vi "UHR-Fleezers Control (host) -Mau_stepping.vi"(0 "Tab Control":T5(tab)) -> ()   [LabVIEW 2013] (continued)
            n1103 = case shown="True" "Move Trap After?" {
              frame False {
              }
              frame True {
                n1104 = property on="Trap Delta (MHz)" class="DigNum (strict)"("Val(Sgnl)"="Dip Trap Delta 2 (MHz)") -> ()  [unwired: 2 in, 2 out]
              }
            }
          }
          frame #3 {
            n1105 = case shown="True" "Green ON After?" {
              frame False {
              }
              frame True {
                n1106 = property on="Green Laser ON/Interlacing" class="Bool (strict)"("Val(Sgnl)"=TRUE ("Value (Signaling)")) -> ()  [unwired: 2 in, 2 out]
              }
            }
          }
          frame #4 {
            n1107 = Wait (ms)(milliseconds to wait=u32 500) -> ()  [unwired: 1 out]
          }
          frame #5 {
            n1108 = case shown="True" "Save Data After?" {
              frame False {
              }
              frame True {
                n1109 = property on="Start Saving" class="Bool (strict)"("Val(Sgnl)"=TRUE ("Value (Signaling)")) -> ()  [unwired: 2 in, 2 out]
              }
            }
          }
        }
      }
      event "Profile": Value Change {
        n1110 = event-data() -> ()  [unwired: 1 in, 5 out]
        n1111 = flat-sequence {
          frame #0 {
            w1714 = 0.0 ("element")
            n1112 = Build Array(w1714, "Y change (mm)", w1714) -> ()  [unwired: 1 out]
          }
          frame #1 {
            # "stop saving"
            n1113 = local write "Stop Saving"(TRUE ("Stop Saving")) -> ()
            n1114 = local write "Stage Moving"(FALSE ("Stage Moving")) -> ()
          }
        }
      }
      event "Got ADig bead": Value Change {
        n1115 = event-data() -> ()  [unwired: 1 in, 5 out]
        n1116 = property on="Move Cap. 1 (DNA Top)" class="Bool (strict)"("Val(Sgnl)"=TRUE ("Value (Signaling)")) -> ()  [unwired: 2 in, 2 out]
        n1117 = property on="Inject Top:" class="Bool (strict)"("Val(Sgnl)"=FALSE ("Value (Signaling)")) -> ()  [unwired: 2 in, 2 out]
      }
      event "Got DNA bead": Value Change {
        n1118 = event-data() -> ()  [unwired: 1 in, 5 out]
        n1119 = property on="Cal/Data Acq. Spot" class="Bool (strict)"("Val(Sgnl)"=TRUE ("Value (Signaling)")) -> ()  [unwired: 2 in, 2 out]
        n1120 = property on="Main:" class="Bool (strict)"("Val(Sgnl)"=FALSE ("Value (Signaling)")) -> ()  [unwired: 2 in, 2 out]
      }
      event "Take Stepping Data": Value Change {
        n1121 = event-data() -> ()  [unwired: 1 in, 5 out]
        n1122 = local read "Save ave N"() -> (w1732:dbl)
        n1123 = flat-sequence {
          tunnel: w1732 -> [w1734]
          tunnel: [w1734] -> w1727
          tunnel: [w1736] -> w1728
          tunnel: w1727 -> [w1736]
          tunnel: [w1738] -> w1729
          tunnel: w1728 -> [w1738]
          tunnel: [w1741] -> w1730
          tunnel: w1729 -> [w1741]
          tunnel: [w1743] -> w1731
          tunnel: w1730 -> [w1743]
          tunnel: [w1745] -> w1725
          tunnel: w1731 -> [w1745]
          tunnel: w1725 -> [w1748]
          tunnel: [w1748] -> w1724
          tunnel: w1724 -> [w1749]
          tunnel: [w1749] -> w1726
          tunnel: w1726 -> [w1755]
          frame #0 {
            n1124 = property on="Save ave N" class="DigNum (strict)"("Val(Sgnl)"="Save ave factor") -> ()  [unwired: 2 in, 2 out]
          }
          frame #1 {
            n1125 = Wait (ms)(milliseconds to wait=u32 100) -> ()  [unwired: 1 out]
          }
          frame #2 {
            n1126 = local read "Offset 2 Start (MHz)"() -> (w1740:dbl)
            n1127 = property on="Saved AOD Raster Scan Parameter Sets" class="Arr (strict)"("Index Values"=u32[] [2]) -> ()  [unwired: 2 in, 2 out]
            n1128 = property on="Trap Delta (MHz)" class="DigNum (strict)"("Val(Sgnl)"=w1740) -> ()  [unwired: 2 in, 2 out]
          }
          frame #3 {
            n1129 = property on="Load parameters" class="Bool (strict)"("Val(Sgnl)"=TRUE ("Value (Signaling)")) -> ()  [unwired: 2 in, 2 out]
          }
          frame #4 {
            n1130 = Wait (ms)(milliseconds to wait=u32 100) -> ()  [unwired: 1 out]
          }
          frame #5 {
            n1131 = property on="Trap Raster Scan" class="Bool (strict)"("Val(Sgnl)"=TRUE ("Value (Signaling)")) -> ()  [unwired: 2 in, 2 out]
          }
          frame #6 {
            n1132 = Wait (ms)(milliseconds to wait=u32 1000) -> ()  [unwired: 1 out]
          }
          frame #7 {
            n1133 = while {
              stop <- w1752 stop-if-true
              n1134 = local read "Raster Scanning..."() -> (w1754:bool)
              n1135 = local read "Saving..."() -> (w1753:bool)
              n1136 = Not(x=w1753) -> (.not. x?=w1750:bool)
              n1137 = Not(x=w1754) -> (.not. x?=w1751:bool)
              n1138 = And(x=w1751, y=w1750) -> (x .and. y?=w1752:bool)
            }
          }
          frame #8 {
            n1139 = property on="Save ave N" class="DigNum (strict)"("Val(Sgnl)"=w1755) -> ()  [unwired: 2 in, 2 out]
          }
        }
      }
      event "Step Size (nm)": Value Change {
        n1140 = event-data() -> ()  [unwired: 1 in, 5 out]
        n1141 = flat-sequence {
          frame #0 {
            n1142 = property on="Saved AOD Raster Scan Parameter Sets" class="Arr (strict)"("Index Values"=u32[] [1]) -> ()  [unwired: 2 in, 2 out]
          }
          frame #1 {
            n1143 = Multiply(x="N Steps", y="Step Size (nm)") -> (x*y=w1757:dbl)
            n1144 = property on="Scan Speed AOD (nm/s) 2" class="DigNum (strict)"("Value"="Step Size (nm)") -> ()  [unwired: 2 in, 2 out]
            n1145 = property on="Step Size AOD (nm) 2" class="DigNum (strict)"("Value"="Step Size (nm)") -> ()  [unwired: 2 in, 2 out]
            n1146 = property on="Scan Range AOD (nm) 2" class="DigNum (strict)"("Value"=w1757) -> ()  [unwired: 2 in, 2 out]
          }
        }
      }
      event "Take Detection Laser\nImage": Value Change {
        n1147 = event-data() -> ()  [unwired: 1 in, 5 out]
        n1148 = flat-sequence {
          tunnel: [w1785] -> w1775
          tunnel: [w1784] -> w1768
          tunnel: [w1783] -> w1760
          tunnel: [w1788] -> w1776
          tunnel: w1775 -> [w1788]
          tunnel: [w1787] -> w1769
          tunnel: w1768 -> [w1787]
          tunnel: [w1786] -> w1761
          tunnel: w1760 -> [w1786]
          tunnel: [w1792] -> w1777
          tunnel: w1776 -> [w1792]
          tunnel: [w1791] -> w1770
          tunnel: w1769 -> [w1791]
          tunnel: [w1790] -> w1762
          tunnel: w1761 -> [w1790]
          tunnel: [w1798] -> w1778
          tunnel: w1777 -> [w1798]
          tunnel: [w1797] -> w1771
          tunnel: w1770 -> [w1797]
          tunnel: [w1796] -> w1763
          tunnel: w1762 -> [w1796]
          tunnel: [w1802] -> w1779
          tunnel: w1778 -> [w1802]
          tunnel: [w1801] -> w1772
          tunnel: w1771 -> [w1801]
          tunnel: [w1800] -> w1764
          tunnel: w1763 -> [w1800]
          tunnel: [w1806] -> w1780
          tunnel: w1779 -> [w1806]
          tunnel: [w1805] -> w1773
          tunnel: w1772 -> [w1805]
          tunnel: [w1804] -> w1765
          tunnel: w1764 -> [w1804]
          tunnel: [w1810] -> w1781
          tunnel: w1780 -> [w1810]
          tunnel: [w1809] -> w1774
          tunnel: w1773 -> [w1809]
          tunnel: [w1808] -> w1766
          tunnel: w1765 -> [w1808]
          tunnel: w1781 -> [w1816]
          tunnel: w1774 -> [w1815]
          tunnel: [w1813] -> w1767
          tunnel: w1766 -> [w1813]
          tunnel: w1767 -> [w1817]
          frame #0 {
            n1149 = local read "Green Laser ON/Interlacing"() -> (w1785:bool)
            n1150 = local read "Green laser mode"() -> (w1784:enum32{"Laser ON", "Laser OFF", "Interlace"})
            n1151 = local read "Green FB On/Off"() -> (w1783:bool)
          }
          frame #1 {
            n1152 = property on="Green FB On/Off" class="Bool (strict)"("Val(Sgnl)"=FALSE ("Value (Signaling)")) -> ()  [unwired: 2 in, 2 out]
          }
          frame #2 {
            n1153 = property on="Green Laser ON/Interlacing" class="Bool (strict)"("Val(Sgnl)"=TRUE ("Value (Signaling)")) -> ()  [unwired: 2 in, 2 out]
            n1154 = property on="Flip Green Filter" class="Bool (strict)"("Val(Sgnl)"=TRUE ("Value (Signaling)")) -> ()  [unwired: 2 in, 2 out]
            n1155 = property on="Green laser mode" class="RadioBtnsControl (strict)"("Val(Sgnl)"=enum32{"Laser ON", "Laser OFF", "Interlace"}."Laser ON" ("Value (Signaling)")) -> ()  [unwired: 2 in, 2 out]
          }
          frame #3 {
            n1156 = Wait (ms)(milliseconds to wait=u32 500) -> ()  [unwired: 1 out]
          }
          frame #4 {
            n1157 = property on="Confocal Image" class="Bool (strict)"("Val(Sgnl)"=TRUE ("Value (Signaling)")) -> ()  [unwired: 2 in, 2 out]
          }
          frame #5 {
            n1158 = Wait (ms)(milliseconds to wait=u32 2000) -> ()  [unwired: 1 out]
          }
          frame #6 {
            n1159 = while {
              stop <- w1811 stop-if-true
              n1160 = local read "Saving..."() -> (w1812:bool)
              n1161 = Not(x=w1812) -> (.not. x?=w1811:bool)
            }
          }
          frame #7 {
            n1162 = property on="Flip Green Filter" class="Bool (strict)"("Val(Sgnl)"=TRUE ("Value (Signaling)")) -> ()  [unwired: 2 in, 2 out]
            n1163 = property on="Green Laser ON/Interlacing" class="Bool (strict)"("Val(Sgnl)"=w1816) -> ()  [unwired: 2 in, 2 out]
            n1164 = property on="Green laser mode" class="RadioBtnsControl (strict)"("Val(Sgnl)"=w1815) -> ()  [unwired: 2 in, 2 out]
          }
          frame #8 {
            n1165 = property on="Green FB On/Off" class="Bool (strict)"("Val(Sgnl)"=w1817) -> ()  [unwired: 2 in, 2 out]
          }
        }
      }
      event "Stop All": Value Change {
        n1166 = event-data() -> ()  [unwired: 1 in, 5 out]
        n1167 = local read "Stop All"() -> (w1818:bool)
      }
    }
    n1168 = node-c288() -> ()  [unwired: 1 in, 1 out]
  }
  n1169 = node-c288() -> (w76:T24)  [unwired: 4 out]
  n1170 = timed-loop "Mouse control: trap position (AOM deflection), set confocal spot from image" {
    tunnel: [w1820] -> w34
    tunnel: w24 -> [w1819]
    timing: w76 -> [_]
    timing-out: [_] -> w75
    stop <- w1820 stop-if-true
    n1171 = node-c288() -> ()  [unwired: 2 out]
    n1172 = event shown="[0] \"Pane\": Mouse Down" {
      selector: _ -> [_ _]
      dyn-events: _ -> [_ _]
      timeout: _ -> [_ _]
      tunnel: w1819 -> [w1823 _]
      event Mouse Down {
        n1173 = event-data() -> ("Time"=w1825:u32, "Coords"=w1824:T8, "Button"=w1826:u16)  [unwired: 6 out]
        n1174 = case shown="1" w1826 {
          tunnel: w1825 -> [_ _ w1929]
          tunnel: w1824 -> [_ w1863 w1927]
          tunnel: w1823 -> [_ _ w1925]
          frame 0, Default {
          }
          frame 1 {
            n1175 = property on="APD 2" class="ImageControl"() -> ("Displayed Image Position"=w1833:cluster{"Left":i32, "Top":i32})  [unwired: 2 in, 2 out]
            n1176 = property on="APD 1" class="ImageControl"() -> ("Displayed Image Position"=w1862:cluster{"Left":i32, "Top":i32})  [unwired: 2 in, 2 out]
            n1177 = property on="Detection Laser X" class="ImageControl"() -> ("Displayed Image Position"=w1859:cluster{"Left":i32, "Top":i32})  [unwired: 2 in, 2 out]
            n1178 = property on="Detection Laser Y" class="ImageControl"() -> ("Displayed Image Position"=w1858:cluster{"Left":i32, "Top":i32})  [unwired: 2 in, 2 out]
            n1179 = property on="APD 2" class="ImageControl"() -> ("Displayed Image Size"=w1832:cluster{"Width":u32, "Height":u32})  [unwired: 2 in, 2 out]
            n1180 = property on="APD 1" class="ImageControl"() -> ("Displayed Image Size"=w1860:cluster{"Width":u32, "Height":u32})  [unwired: 2 in, 2 out]
            n1181 = property on="Detection Laser X" class="ImageControl"() -> ("Displayed Image Size"=w1861:cluster{"Width":u32, "Height":u32})  [unwired: 2 in, 2 out]
            n1182 = property on="Detection Laser Y" class="ImageControl"() -> ("Displayed Image Size"=w1857:cluster{"Width":u32, "Height":u32})  [unwired: 2 in, 2 out]
            n1183 = Unbundle By Name(w1832) -> ("Width"=w1829:u32, "Height"=w1828:u32)
            n1184 = Unbundle By Name(w1833) -> ("Left"=w1831:i32, "Top"=w1830:i32)
            n1185 = Unbundle By Name(w1860) -> ("Width"=w1854:u32, "Height"=w1853:u32)
            n1186 = Unbundle By Name(w1861) -> ("Width"=w1850:u32, "Height"=w1849:u32)
            n1187 = Unbundle By Name(w1857) -> ("Width"=w1846:u32, "Height"=w1845:u32)
            n1188 = Unbundle By Name(w1862) -> ("Left"=w1856:i32, "Top"=w1855:i32)
            n1189 = Unbundle By Name(w1859) -> ("Left"=w1852:i32, "Top"=w1851:i32)
            n1190 = Unbundle By Name(w1858) -> ("Left"=w1848:i32, "Top"=w1847:i32)
            n1191 = Bundle("Left"=w1831, "Top"=w1830, "Width"=w1829, "Height"=w1828) -> (w1827:T33)  [unwired: 1 in]
            n1192 = Bundle("Left"=w1856, "Top"=w1855, "Width"=w1854, "Height"=w1853) -> (w1844:T33)  [unwired: 1 in]
            n1193 = Bundle("Left"=w1852, "Top"=w1851, "Width"=w1850, "Height"=w1849) -> (w1843:T33)  [unwired: 1 in]
            n1194 = Bundle("Left"=w1848, "Top"=w1847, "Width"=w1846, "Height"=w1845) -> (w1842:T33)  [unwired: 1 in]
            n1195 = Build Cluster Array(w1827, w1844, w1843, w1842) -> (w1841:T34)
            n1196 = for {
              tunnel: w1863 -> [w1874]
              tunnel: w1841 -> [w1875] mode=indexing
              shift-right: [w1872] -> w1839
              shift-left: TRUE -> [w1873]
              shift-right: [w1871] -> w1837
              shift-left: _ -> [w1867]
              shift-right: [w1870] -> w1836
              shift-left: _ -> [w1866]
              shift-right: [w1869] -> w1835
              shift-left: _ -> [w1865]
              shift-right: [w1868] -> w1834
              shift-left: _ -> [w1864]
              n1197 = case shown="True" w1873 {
                selector: w1873 -> [w1880 _]
                tunnel: w1875 -> [_ w1889]
                tunnel: w1874 -> [_ w1887]
                tunnel: [w1880 w1885] -> w1872
                tunnel: [w1879 w1884] -> w1871
                tunnel: [w1878 w1883] -> w1870
                tunnel: [w1877 w1882] -> w1869
                tunnel: [w1876 w1881] -> w1868
                tunnel: w1867 -> [w1879 _]
                tunnel: w1866 -> [w1878 _]
                tunnel: w1865 -> [w1877 _]
                tunnel: w1864 -> [w1876 _]
                frame False {
                }
                frame True {
                  n1198 = Unbundle(w1889) -> (w1888:T33)
                  n1199 = call "isclickinwindow.vi"("Image Param"=w1888, "Point32"=w1887) -> ("4 Y"=w1881:i32, "3 Height"=w1882:i32, "2 X"=w1883:i32, "1 Width"=w1884:i32, "In image?"=w1886:bool)  [unwired: 1 in]
                  n1200 = Not(x=w1886) -> (.not. x?=w1885:bool)
                }
              }
            }
            n1201 = Not(x=w1839) -> (.not. x?=w1838:bool)
            n1202 = case shown="True" w1838 {
              tunnel: w1836 -> [_ w1902]
              tunnel: w1834 -> [_ w1901]
              tunnel: w1837 -> [_ w1900]
              tunnel: w1835 -> [_ w1899]
              frame False {
              }
              frame True {
                w1895 = FALSE ("Get Point")
                n1203 = local read "Scan lines (y)"() -> (w1904:u64)
                n1204 = local read "Actual MCL Inc (V)"() -> (w1896:dbl)
                n1205 = local read "Scan steps (MCL)"() -> (w1903:u64)
                n1206 = Divide "Y Pix/step"(x=w1899, y=w1904) -> (x/y=w1911:dbl)
                n1207 = Divide "Y V/pix"(x=w1896, y=w1911) -> (x/y=w1910:dbl)
                n1208 = Divide "Y half step offset"(x=w1896, y=2.0) -> (x/y=w1912:dbl)
                n1209 = Divide "X pix/step"(x=w1900, y=w1903) -> (x/y=w1909:dbl)
                n1210 = Negate(x=w1912) -> (-x=w1913:dbl)
                n1211 = local read "Initial Y"() -> (w1919:dbl)
                n1212 = Multiply(x=w1901, y=w1910) -> (x*y=w1920:dbl)
                n1213 = Divide "X half step offset"(x=w1896, y=2.0) -> (x/y=w1906:dbl)
                n1214 = Divide "X V/pix"(x=w1896, y=w1909) -> (x/y=w1908:dbl)
                n1215 = Multiply(x=w1896, y=w1903) -> (x*y=w1915:dbl)
                n1216 = Compound Arithmetic op=ADD(w1913, w1920, w1919) -> (w1897:dbl)
                "Pointer Y (V)" <- w1897
                n1217 = Multiply(x=w1908, y=w1902) -> (x*y=w1917:dbl)
                n1218 = Negate(x=w1906) -> (-x=w1905:dbl)
                n1219 = local read "Initial X"() -> (w1918:dbl)
                n1220 = Negate(x=w1917) -> (-x=w1916:dbl)
                n1221 = Compound Arithmetic op=ADD(w1905, w1915, w1918, w1916) -> (w1898:dbl)
                "Pointer X (V)" <- w1898
                n1222 = Or(x="Set X Only", y="Set Confocal Spot (X-Y)") -> (x .or. y?=w1891:bool)
                n1223 = Or(x="Set Confocal Spot (X-Y)", y="Set Y Only") -> (x .or. y?=w1890:bool)
                n1224 = case shown="True" w1891 {
                  tunnel: w1898 -> [_ w1921]
                  frame False {
                  }
                  frame True {
                    n1225 = property on="AO2" class="Slide (strict)"("Val(Sgnl)"=w1921) -> ()  [unwired: 2 in, 2 out]
                  }
                }
                n1226 = case shown="True" w1890 {
                  tunnel: w1897 -> [_ w1922]
                  frame False {
                  }
                  frame True {
                    n1227 = property on="AO1" class="Slide (strict)"("Val(Sgnl)"=w1922) -> ()  [unwired: 2 in, 2 out]
                  }
                }
                n1228 = local write "Set Confocal Spot (X-Y)"(w1895) -> ()
                n1229 = local write "Set X Only"(w1895) -> ()
                n1230 = local write "Set Y Only"(w1895) -> ()
              }
            }
          }
          frame 3 {
            n1231 = local read "BD 2 Frequency 1 (MHz)"() -> (w1923:dbl)
            n1232 = local read "BD 1 Frequency 1 (MHz)"() -> (w1924:dbl)
            n1233 = local write "Manipulating Trap"(TRUE ("Manipulating Trap")) -> ()
            n1234 = local write "Coords"(T8 {"Horizontal"=0, "Vertical"=0} ("Coords")) -> ()
            n1235 = while {
              tunnel: w1929 -> [w1934]
              tunnel: w1927 -> [w1933]
              tunnel: w1925 -> [w1932]
              tunnel: w1924 -> [w1931]
              tunnel: w1923 -> [w1930]
              stop <- w1935 stop-if-true
              n1236 = event shown="[0] \"Pane\": Mouse Move" {
                selector: _ -> [_ _]
                dyn-events: _ -> [_ _]
                timeout: _ -> [_ _]
                tunnel: ["Force Manip Abort" w1999] -> w1935
                tunnel: w1934 -> [w1942 _]
                tunnel: w1933 -> [w1940 _]
                tunnel: w1932 -> [w1939 _]
                tunnel: w1931 -> [w1938 _]
                tunnel: w1930 -> [w1937 _]
                event Mouse Move {
                  n1237 = event-data() -> ("Time"=w1943:u32, "Coords"=w1944:T8)  [unwired: 3 out]
                  n1238 = Less?(x=w1943, y=w1942) -> (x < y?=w1941:bool)
                  n1239 = case "Makes sure old motion events prior to mouse click aren't used" shown="False" w1941 {
                    tunnel: w1944 -> [w1986 _]
                    tunnel: w1940 -> [w1987 _]
                    tunnel: w1939 -> [w1964 _]
                    tunnel: w1938 -> [w1960 _]
                    tunnel: w1937 -> [w1959 _]
                    frame False {
                      n1240 = Subtract(x=w1986, y=w1987) -> (x-y=w1985:T8)
                      "Coords" <- w1985
                      n1241 = local read "Y RF Frequency Limits (MHz)"() -> (w1945:T16)
                      n1242 = To Double Precision Float(number=w1985) -> (double precision float=w1984:cluster{"Horizontal":dbl, "Vertical":dbl})
                      n1243 = Multiply(x=cluster{"Horizontal":dbl, "Vertical":dbl} {"Horizontal"=-1.0, "Vertical"=1.0}, y="Manipulation Scaling") -> (x*y=w1980:cluster{"Horizontal":dbl, "Vertical":dbl})
                      n1244 = local read "X RF Frequency Limits (MHz)"() -> (w1946:T16)
                      n1245 = Multiply(x=w1984, y=w1980) -> (x*y=w1982:cluster{"Horizontal":dbl, "Vertical":dbl})
                      n1246 = Unbundle By Name(w1982) -> ("Horizontal"=w1977:dbl, "Vertical"=w1981:dbl)
                      n1247 = Unbundle By Name(w1945) -> ("Maximum"=w1948:dbl, "Minimum"=w1947:dbl)
                      n1248 = Boolean To (0,1)(Boolean="Manip. X?") -> (0, 1=w1975:i16)
                      n1249 = Boolean To (0,1)(Boolean="Manip. Y?") -> (0, 1=w1972:i16)
                      n1250 = local read "BD 1 Frequency 2 (MHz)"() -> (w1962:dbl)
                      n1251 = Multiply(x=w1981, y=w1972) -> (x*y=w1974:dbl)
                      n1252 = Multiply(x=w1975, y=w1977) -> (x*y=w1978:dbl)
                      n1253 = local read "BD 2 Frequency 2 (MHz)"() -> (w1961:dbl)
                      n1254 = Unbundle By Name(w1946) -> ("Maximum"=w1950:dbl, "Minimum"=w1949:dbl)
                      n1255 = Add(x=w1959, y=w1974) -> (x+y=w1952:dbl)
                      n1256 = Add(x=w1960, y=w1978) -> (x+y=w1954:dbl)
                      n1257 = In Range and Coerce(upper limit=w1950, x=w1954, lower limit=w1949) -> (coerced(x)=w1953:dbl)  [unwired: 1 out]
                      n1258 = In Range and Coerce(upper limit=w1948, x=w1952, lower limit=w1947) -> (coerced(x)=w1951:dbl)  [unwired: 1 out]
                      n1259 = Subtract(x=w1953, y=w1962) -> (x-y=w1971:dbl)
                      n1260 = Subtract(x=w1951, y=w1961) -> (x-y=w1970:dbl)
                      n1261 = Square(x=w1971) -> (x^2=w1969:dbl)
                      n1262 = Square(x=w1970) -> (x^2=w1968:dbl)
                      n1263 = Add(x=w1969, y=w1968) -> (x+y=w1967:dbl)
                      n1264 = Square Root(x=w1967) -> (sqrt(x)=w1963:dbl)
                      n1265 = In Range and Coerce(upper limit="Limit Max (MHz)", x=w1963, lower limit="Limit Min (MHz)") -> (In Range?=w1956:bool)  [unwired: 1 out]
                      n1266 = Not(x="Limits Enable") -> (.not. x?=w1955:bool)
                      n1267 = Or(x=w1956, y=w1955) -> (x .or. y?=w1957:bool)
                      n1268 = case shown="True" w1957 {
                        tunnel: w1964 -> [_ w1997]
                        tunnel: w1963 -> [_ w1988]
                        tunnel: w1953 -> [_ w1995]
                        tunnel: w1962 -> [_ w1994]
                        tunnel: w1951 -> [_ w1993]
                        tunnel: w1961 -> [_ w1992]
                        tunnel: w1946 -> [_ w1990]
                        tunnel: w1945 -> [_ w1989]
                        frame False {
                        }
                        frame True {
                          n1269 = local read "BD 1 Frequency 3 (MHz)"() -> (w1996:dbl)
                          n1270 = local read "BD 2 Frequency 3 (MHz)"() -> (w1991:dbl)
                          n1271 = local write "Trap Delta (MHz)"(w1988) -> ()
                          n1272 = property on="Initial delta (MHz)" class="DigNum (strict)"("Val(Sgnl)"=w1988) -> ()  [unwired: 2 in, 2 out]
                          n1273 = call "set RF board frequency - interlace.vi"("Board 2 Frequency Limits"=w1989, "Board 1 Frequency Limits"=w1990, "FPGA VI Reference In"=w1997, "Board 2 Frequency 3 (MHz)"=w1991, "Board 1 Frequency 3 (MHz)"=w1996, "Board 2 Frequency 2 (MHz)"=w1992, "Board 2 Frequency 1 (MHz)"=w1993, "Board 1 Frequency 2 (MHz)"=w1994, "Board 1 Frequency 1  (MHz)"=w1995) -> ()  [unwired: 1 in, 2 out]
                          n1274 = local write "BD 2 Frequency 1 (MHz)"(w1993) -> ()
                          n1275 = local write "BD 1 Frequency 1 (MHz)"(w1995) -> ()
                        }
                      }
                    }
                    frame True {
                    }
                  }
                }
                event Mouse Up {
                  n1276 = event-data() -> ("Button"=w1998:u16)  [unwired: 8 out]
                  n1277 = case shown="3" w1998 {
                    tunnel: [FALSE TRUE] -> w1999
                    frame 0, Default {
                    }
                    frame 3 {
                      n1278 = local write "Manipulating Trap"(FALSE ("Manipulating Trap")) -> ()
                    }
                  }
                }
              }
            }
          }
        }
      }
      event Mouse Move {
        n1279 = event-data() -> ()  [unwired: 6 out]
      }
    }
    n1280 = local read "Stop All"() -> (w1820:bool)
    n1281 = node-c288() -> ()  [unwired: 2 out]
  }
  n1282 = node-c288(w14) -> ()  [unwired: 1 out]
  n1283 = node-c288(w68) -> ()  [unwired: 1 out]
  n1284 = node-c288(w75) -> ()  [unwired: 1 out]
  n1285 = node-c288(i64 1 ("Period"), 1 ("Processor")) -> (w164:T24)  [unwired: 2 out]
  n1286 = timed-loop "Acquire Data" {
    tunnel: w24 -> [w2268]
    tunnel: w40 -> [w2267]
    tunnel: [w2298] -> w33
    tunnel: [w2292] -> w32
    timing: w164 -> [_]
    timing-out: [_] -> w163
    tunnel: w59 -> [w2097]
    stop <- "Stop All" stop-if-true
    (unwired) u32 0 ("Number of Elements")
    w2084 = "NI_ChannelName" ("name")
    n1287 = node-c288() -> ()  [unwired: 2 out]
    n1288 = First Call?() -> (First Call?: T/F=w2050:bool)
    n1289 = Or(x="Reset", y=w2050) -> (x .or. y?=w2051:bool)
    n1290 = case "Reset data stream" shown="True" w2051 {
      tunnel: w2268 -> [w2314 w2322]
      tunnel: w2267 -> [w2313 w2321]
      tunnel: [w2314 w2316] -> w2263
      tunnel: [w2313 w2315] -> w2262
      frame False {
      }
      frame True {
        w2319 = TRUE ("AI to FIFO")
        n1291 = local write "Overflow (data lost)"(FALSE ("Overflow (data lost)")) -> ()
        n1292 = call "reset FPGA DMA.vi"("error in"=w2321, "FPGA VI Reference In"=w2322) -> ("error out"=w2317:errorcluster, "FPGA VI Reference Out"=w2318:T19)
        n1293 = xnode "Read/Write Control"("FPGA VI Reference In"=w2318, "error in"=w2317, "AI to FIFO"=w2319, "APD to FIFO"=w2319) -> ("FPGA VI Reference Out"=w2316:T19, "error out"=w2315:errorcluster)
      }
    }
    n1294 = Or(x="Start AOD Scan", y="Trap Raster Scan") -> (x .or. y?=w2213:bool)
    n1295 = case "Start AOM raster scan" shown="True" w2213 {
      tunnel: w2263 -> [w3051 w3061]
      tunnel: w2262 -> [w3050 w3060]
      tunnel: [w3051 w3054] -> w2261
      tunnel: [w3050 w3053] -> w2260
      frame False {
      }
      frame True {
        n1296 = case shown="True" "Restart DMA? (AOD)" {
          tunnel: [w3099 w3101] -> w3055
          tunnel: [w3098 w3100] -> w3056
          tunnel: w3061 -> [w3099 w3103]
          tunnel: w3060 -> [w3098 w3102]
          frame False {
          }
          frame True {
            n1297 = local write "Overflow (data lost)"(FALSE ("Overflow (data lost)")) -> ()
            n1298 = call "reset FPGA DMA.vi"("error in"=w3102, "FPGA VI Reference In"=w3103) -> ("error out"=w3100:errorcluster, "FPGA VI Reference Out"=w3101:T19)
          }
        }
        n1299 = local write "Trap Raster Scan"(FALSE ("Trap Raster Scan")) -> ()
        n1300 = case shown="True" "Move MCL Also?" {
          tunnel: w3056 -> [w3064 w3093]
          tunnel: w3055 -> [w3065 w3094]
          tunnel: [w3063 w3097] -> w3054
          tunnel: [w3062 w3096] -> w3053
          frame False {
            w3066 = TRUE ("AI to FIFO")
            n1301 = xnode "Read/Write Control"("FPGA VI Reference In"=w3065, "error in"=w3064, "AI to FIFO"=w3066, "APD to FIFO"=w3066, "Start scan"=w3066) -> ("FPGA VI Reference Out"=w3063:T19, "error out"=w3062:errorcluster)
          }
          frame True {
            w3090 = FALSE ("1D or 2D Scan?")
            w3095 = TRUE ("AI to FIFO")
            # "Count for MCL loop"
            # "N total cycles"
            # "N steps"
            # "V_int"
            n1302 = local read "Scan Range (nm)"() -> (w3072:dbl)
            n1303 = local read "Number of F/B Scans (AOD)"() -> (w3089:u16)
            n1304 = Sign(1:w3072) -> (0:w3071:dbl)
            n1305 = Compound Arithmetic op=MULTIPLY(w3072, "MCL Step Position Ratio", "MCL/AOM Scale Tweak") -> (w3076:dbl)
            n1306 = Negate(x=w3071) -> (-x=w3068:dbl)
            n1307 = Multiply(x=w3068, y="MCL Step Increment (V_int)") -> (x*y=w3070:dbl)
            n1308 = Divide(x=w3076, y="MCL X Cal (nm/V)") -> (x/y=w3082:dbl)
            n1309 = Multiply(x=32767.0 ("y"), y=w3082) -> (x*y=w3088:dbl)
            n1310 = local read "Total Counts (ticks)"() -> (w3073:u32)
            n1311 = local read "Cycles/step (AOD)"() -> (w3084:u64)
            n1312 = local read "Scan steps (AOD)"() -> (w3085:u64)
            n1313 = Divide(x=w3088, y=10.0) -> (x/y=w3081:dbl)
            n1314 = Divide(x=w3081, y="MCL Step Increment (V_int)") -> (x/y=w3079:dbl)
            n1315 = Absolute Value(x=w3079) -> (abs(x)=w3067:dbl)
            n1316 = Compound Arithmetic op=MULTIPLY(w3085, w3084, w3073) -> (w3080:u64)
            n1317 = local write "wait to reset values"(w3095) -> ()
            n1318 = local write "MCL Scanning"(w3095) -> ()
            n1319 = Divide(x=w3080, y=w3067) -> (x/y=w3077:dbl)
            "MCL Count" <- w3077
            n1320 = xnode "Read/Write Control"("FPGA VI Reference In"=w3094, "error in"=w3093, "Scan steps (MCL)"=w3067, "Number of scans (MCL)"=w3089, "Cycles per step (MCL)"=u64 1, "Scan freq.  increment (MCL)"=w3070, "1D or 2D Scan?"=w3090, "MCL Scan Axis"=w3090, "Cont. Scan (MCL)"=w3090, "MCL count"=w3077) -> ("FPGA VI Reference Out"=w3092:T19, "error out"=w3091:errorcluster)
            n1321 = xnode "Read/Write Control"("FPGA VI Reference In"=w3092, "error in"=w3091, "AI to FIFO"=w3095, "APD to FIFO"=w3095, "Start scan"=w3095, "Start scan (MCL)"=w3095) -> ("FPGA VI Reference Out"=w3097:T19, "error out"=w3096:errorcluster)
          }
        }
        "Raster Scanning..." <- TRUE ("Scanning...")
      }
    }
    n1322 = And(x="Save scans", y=w2213) -> (x .and. y?=w2259:bool)
    n1323 = Compound Arithmetic op=OR("Start MCL Scan", "Confocal Image", "Confocal Linescan") -> (w2211:bool)
    n1324 = And(x="Save Data (MCL)", y=w2211) -> (x .and. y?=w2258:bool)
    n1325 = case "Start MCL raster scan" shown="True" w2211 {
      tunnel: w2261 -> [w2605 w2620]
      tunnel: w2260 -> [w2604 w2619]
      tunnel: [w2605 w2615] -> w2019
      tunnel: [w2604 w2614] -> w2018
      tunnel: [FALSE w2613] -> w2244
      tunnel: "Start MCL Scan" -> [_ w2608]
      tunnel: "Confocal Image" -> [_ w2607]
      tunnel: "Confocal Linescan" -> [_ _]
      frame False {
      }
      frame True {
        w2613 = TRUE
        n1326 = case shown="True" "Restart DMA? (MCL)" {
          tunnel: [w2665 w2667] -> w2618
          tunnel: [w2664 w2666] -> w2617
          tunnel: w2620 -> [w2665 w2670]
          tunnel: w2619 -> [w2664 w2669]
          frame False {
          }
          frame True {
            n1327 = call "reset FPGA DMA.vi"("error in"=w2669, "FPGA VI Reference In"=w2670) -> ("error out"=w2666:errorcluster, "FPGA VI Reference Out"=w2667:T19)
            n1328 = local write "Overflow (data lost)"(FALSE ("Overflow (data lost)")) -> ()
          }
        }
        n1329 = case shown="False" w2608 {
          selector: w2608 -> [_ w2624]
          tunnel: w2607 -> [w2623 _]
          tunnel: [w2623 w2624] -> w2606
          frame False {
            n1330 = property on="2D or 1D Scan" class="Bool (strict)"("Val(Sgnl)"=w2623) -> ()  [unwired: 2 in, 2 out]
            n1331 = property on="Confocal Image" class="Bool (strict)"("Value"=FALSE ("Start Confocal Map")) -> ()  [unwired: 2 in, 2 out]
          }
          frame True {
          }
        }
        n1332 = local write "MCL Scanning"(w2613) -> ()
        n1333 = local read "AO1"() -> (w2610:dbl)
        n1334 = local read "AO2"() -> (w2609:dbl)
        n1335 = case shown="True" "Center Scan" {
          tunnel: w2618 -> [w2631 w2663]
          tunnel: w2617 -> [w2630 w2662]
          tunnel: [w2629 w2661] -> w2615
          tunnel: [w2628 w2660] -> w2614
          tunnel: [w2626 w2647] -> w2612
          tunnel: [w2625 w2646] -> w2611
          tunnel: w2610 -> [w2626 w2652]
          tunnel: w2609 -> [w2625 w2655]
          tunnel: w2606 -> [_ _]
          frame False {
            w2627 = TRUE ("AI to FIFO")
            n1336 = xnode "Read/Write Control"("FPGA VI Reference In"=w2631, "error in"=w2630, "AI to FIFO"=w2627, "APD to FIFO"=w2627, "Start scan (MCL)"=w2627) -> ("FPGA VI Reference Out"=w2629:T19, "error out"=w2628:errorcluster)
          }
          frame True {
            w2659 = TRUE ("AI to FIFO")
            n1337 = local read "Scan steps (MCL)"() -> (w2638:u64)
            n1338 = local read "Scan lines (y)"() -> (w2634:u64)
            n1339 = local read "Fast Scan Dir"() -> (w2645:bool)
            n1340 = local read "Actual MCL Inc (V)"() -> (w2635:dbl)
            n1341 = Decrement(x=w2634) -> (x-1=w2633:u64)
            n1342 = Decrement(x=w2638) -> (x-1=w2637:u64)
            n1343 = Multiply(x=w2635, y=w2633) -> (x*y=w2632:dbl)
            n1344 = Divide(x=w2632, y=2.0) -> (x/y=w2642:dbl)
            n1345 = Multiply(x=w2635, y=w2637) -> (x*y=w2636:dbl)
            n1346 = Divide(x=w2636, y=2.0) -> (x/y=w2641:dbl)
            n1347 = Select(t=w2641, s=w2645, f=w2642) -> (s? t:f=w2640:dbl)
            n1348 = Select(t=w2642, s=w2645, f=w2641) -> (s? t:f=w2644:dbl)
            n1349 = Subtract(x=w2652, y=w2644) -> (x-y=w2643:dbl)
            n1350 = Subtract(x=w2655, y=w2640) -> (x-y=w2639:dbl)
            n1351 = local read "2D or 1D Scan"() -> (w2657:bool)
            n1352 = Not(x=w2645) -> (.not. x?=w2651:bool)
            n1353 = Not(x=w2657) -> (.not. x?=w2653:bool)
            n1354 = And(x=w2645, y=w2653) -> (x .and. y?=w2654:bool)
            n1355 = And(x=w2653, y=w2651) -> (x .and. y?=w2656:bool)
            n1356 = Select(t=w2655, s=w2656, f=w2639) -> (s? t:f=w2646:dbl)
            n1357 = Select(t=w2652, s=w2654, f=w2643) -> (s? t:f=w2647:dbl)
            n1358 = call "Volt to I16.vi"("Voltage In"=w2647) -> ("I16 Voltage Out"=w2650:i16)
            n1359 = call "Volt to I16.vi"("Voltage In"=w2646) -> ("I16 Voltage Out"=w2649:i16)
            n1360 = xnode "Read/Write Control"("FPGA VI Reference In"=w2663, "error in"=w2662, "AI to FIFO"=w2659, "APD to FIFO"=w2659, "Start scan (MCL)"=w2659, "AO1"=w2650, "AO2"=w2649) -> ("FPGA VI Reference Out"=w2661:T19, "error out"=w2660:errorcluster)
          }
        }
        "Initial Y" <- w2612
        "Initial X" <- w2611
        "wait to reset values" <- w2613
      }
    }
    n1361 = local read "Trap Pos Elements/DMA read"() -> (w2093:u32)
    n1362 = local read "Trap AI Elements/DMA read"() -> (w2017:u32)
    n1363 = local read "APD Elements/DMA read"() -> (w2136:u32)
    n1364 = local read "Trap AI FIFO Depth"() -> (w2308:u32)
    n1365 = xnode "Invoke Method"("FPGA VI Reference In"=w2019, "error in"=w2018, "Number of Elements"=w2093, "Timeout (ms)"=-1) -> ("Data"=w2057:u16[], "Elements Remaining"=→"Trap Pos FIFO El Remaining":u32)  [unwired: 2 out]
    n1366 = xnode "Invoke Method"("FPGA VI Reference In"=w2019, "error in"=w2018, "Number of Elements"=w2017, "Timeout (ms)"=-1 ("Timeout")) -> ("FPGA VI Reference Out"=w2021:T19, "error out"=w2020:errorcluster, "Data"=w2016:i16[], "Elements Remaining"=w2022:u32)
    "Trap AI FIFO El. Rem." <- w2022
    n1367 = xnode "Get APD Data"("FPGA VI Reference In"=w2019, "error in"=w2018, "Number of Elements"=w2136, "Timeout (ms)"=-1) -> ("Data"=w2135:u32[], "Elements Remaining"=→"APD FIFO Elements Remaining":u32)  [unwired: 2 out]
    n1368 = Subtract(x=w2308, y=w2017) -> (x-y=w2307:u32)
    n1369 = Decimate 1D Array(w2057) -> (w2054:u16[], w2056:u16[], w2055:u16[])
    n1370 = Divide(x=w2022, y=w2307) -> (x/y=w2306:dbl)
    "Buffer Status" <- w2306
    n1371 = To Unsigned Long Integer(number=w2054) -> (unsigned 32bit integer=w2053:u32[])
    n1372 = Join Numbers(hi=w2056, lo=w2055) -> ((hi.lo)=w2052:u32[])
    n1373 = Equal?(x=w2306, y=1.0) -> (x = y?=w2304:bool)
    n1374 = Join Numbers(hi=w2053, lo=w2052) -> ((hi.lo)=w2046:u64[])
    n1375 = call "IR AOM word to freq - vec.vi"("Frequency Word In (double vec)"=w2046) -> ("Frequency Out"=w2092:dbl[])
    n1376 = case "Alert buffer overflow" shown="False" w2304 {
      frame False {
      }
      frame True {
        n1377 = call <vilib>:"Beep.vi"() -> ()  [unwired: 3 in, 9 out]
        "Overflow (data lost)" <- TRUE ("Overflow (data lost)")
      }
    }
    n1378 = Decimate 1D Array(w2092) -> (w2091:dbl[], w2090:dbl[])
    n1379 = Array Size(array=w2016) -> (size(s)=→"Waveform Chart":i32)
    n1380 = Build Array(w2091, w2090) -> (w2089:dbl[][])
    n1381 = local read "Trap Sets"() -> (w2173:u32)
    n1382 = case "Deinterlace trap data, average down PSD" shown="2" w2173 {
      tunnel: w2016 -> [w2700 w2765]
      tunnel: [w2697 w2762] -> w2166
      tunnel: [w2700 w2764] -> w2049
      tunnel: "Detector Type" -> [w2699 w2760]
      tunnel: [w2698 w2763] -> w2165
      tunnel: [w2696 w2761] -> w2279
      frame 1, Default {
        n1383 = Divide(x=w2700, y=3276.7) -> (x/y=w2701:dbl[])
        n1384 = Decimate 1D Array(w2701) -> (w2710:dbl[], w2709:dbl[], w2708:dbl[], w2707:dbl[], w2706:dbl[], w2705:dbl[], w2704:dbl[], w2703:dbl[])
        n1385 = case shown="\"IR-QPD + PSD + FB-QPD position\"" w2699 {
          tunnel: w2710 -> [w2734 w2759]
          tunnel: w2709 -> [w2733 w2758]
          tunnel: w2708 -> [w2718 w2736]
          tunnel: w2707 -> [w2719 w2746]
          tunnel: w2706 -> [w2732 w2757]
          tunnel: w2705 -> [w2731 w2756]
          tunnel: w2704 -> [w2715 w2737]
          tunnel: w2703 -> [w2714 w2735]
          tunnel: [w2713 w2743] -> w2698
          tunnel: [w2712 w2742] -> w2697
          tunnel: [w2711 w2741] -> w2696
          frame "IR-QPD + PSD + FB-QPD", Default {
            w2711 = 0  # Channel pattern
            n1386 = Divide(x=w2734, y=w2719) -> (x/y=w2721:dbl[])
            n1387 = Divide(x=w2733, y=w2719) -> (x/y=w2720:dbl[])
            n1388 = Divide(x=w2732, y=w2715) -> (x/y=w2717:dbl[])
            n1389 = Divide(x=w2731, y=w2714) -> (x/y=w2716:dbl[])
            n1390 = Build Array(w2721, w2720, w2719, w2718, w2717, w2716, w2715, w2714) -> (w2712:dbl[][])
            n1391 = Bundle("T1 Y", "T1 X", "T1 Sum", "FB Sum", "PSD Y", "PSD X", "PSD Y Sum", "PSD X Sum") -> (w2730:T41)  [unwired: 1 out]
            n1392 = Cluster To Array(cluster=w2730) -> (array=w2713:string[])
          }
          frame "IR-QPD + PSD + FB-QPD position" {
            w2741 = 3  # Channel pattern
            n1393 = Negate(x=w2737) -> (-x=w2738:dbl[])
            n1394 = Divide(x=w2759, y=w2746) -> (x/y=w2748:dbl[])
            n1395 = Divide(x=w2758, y=w2746) -> (x/y=w2747:dbl[])
            n1396 = Divide(x=w2757, y=w2737) -> (x/y=w2745:dbl[])
            n1397 = Divide(x=w2756, y=w2738) -> (x/y=w2744:dbl[])
            n1398 = Build Array(w2748, w2747, w2746, w2735, w2736, w2745, w2744, w2737) -> (w2742:dbl[][])
            n1399 = Bundle("T1 Y", "T1 X", "T1 Sum", "FB X", "FB Sum", "PSD Y", "PSD X", "PSD Y Sum") -> (w2755:T41)  [unwired: 1 out]
            n1400 = Cluster To Array(cluster=w2755) -> (array=w2743:string[])
          }
        }
      }
      frame 2 {
        n1401 = case shown="\"UCB Fleezers 052511\"" w2760 {
          tunnel: w2765 -> [w2827 w2894 w2922 w3029]
          tunnel: [w2766 w2886 w2917 w2960] -> w2764
          tunnel: [w2793 w2877 w2919 w3007] -> w2763
          tunnel: [w2792 w2841 w2896 w2974] -> w2762
          tunnel: [w2786 w2876 w2959 w3005] -> w2761
          frame "IR-QPD + PSD + FB-QPD", Default {
            w2786 = 1  # Channel pattern
            # "time average x2 the 4th signal and the 4 psd signals (detection laser)"
            # "deinterlace 3 signals from qpd"
            n1402 = Decimate 1D Array(w2827) -> (w2826:i16[], w2825:i16[], w2791:i16[], w2824:i16[], w2814:i16[], w2812:i16[], w2811:i16[], w2809:i16[])
            n1403 = call "downsample 1D array - double.vi"("Ave N"=2.0, "Array In"=w2814) -> ("Array Out"=w2813:dbl[])  [unwired: 1 out]
            n1404 = call "downsample 1D array - double.vi"("Ave N"=2.0, "Array In"=w2809) -> ("Array Out"=w2808:dbl[])  [unwired: 1 out]
            n1405 = call "downsample 1D array - double.vi"("Ave N"=2.0, "Array In"=w2811) -> ("Array Out"=w2810:dbl[])  [unwired: 1 out]
            n1406 = call "downsample 1D array - double.vi"("Ave N"=2.0, "Array In"=w2812) -> ("Array Out"=w2794:dbl[])  [unwired: 1 out]
            n1407 = Decimate 1D Array(w2826) -> (w2823:i16[], w2795:i16[])
            n1408 = Decimate 1D Array(w2825) -> (w2822:i16[], w2820:i16[])
            n1409 = Decimate 1D Array(w2824) -> (w2821:i16[], w2819:i16[])
            n1410 = Decimate 1D Array(w2791) -> (w2790:i16[], w2789:i16[])
            n1411 = Interleave 1D Arrays(w2823, w2822, w2821, w2795, w2820, w2819, w2790, w2789, w2813, w2794, w2810, w2808) -> (w2807:dbl[])
            n1412 = To Word Integer(number=w2807) -> (16bit integer=w2766:i16[])
            n1413 = Divide(x=w2807, y=3276.7) -> (x/y=w2806:dbl[])
            n1414 = Decimate 1D Array(w2806) -> (w2805:dbl[], w2804:dbl[], w2803:dbl[], w2802:dbl[], w2801:dbl[], w2800:dbl[], w2788:dbl[], w2787:dbl[], w2799:dbl[], w2798:dbl[], w2797:dbl[], w2796:dbl[])
            n1415 = Divide(x=w2805, y=w2803) -> (x/y=w2773:dbl[])
            n1416 = Divide(x=w2804, y=w2803) -> (x/y=w2772:dbl[])
            n1417 = Divide(x=w2802, y=w2800) -> (x/y=w2771:dbl[])
            n1418 = Divide(x=w2801, y=w2800) -> (x/y=w2770:dbl[])
            n1419 = Divide(x=w2799, y=w2797) -> (x/y=w2769:dbl[])
            n1420 = Divide(x=w2798, y=w2796) -> (x/y=w2768:dbl[])
            n1421 = Bundle("T1 Y", "T1 X", "T1 Sum", "T2 Y", "T2 X", "T2 Sum", "T1 FB Sum", "T2 FB Sum", "PSD Y", "PSD X", "PSD Y Sum", "PSD X Sum") -> (w2774:T42)  [unwired: 1 out]
            n1422 = Build Array(w2773, w2772, w2803, w2771, w2770, w2800, w2788, w2787, w2769, w2768, w2797, w2796) -> (w2792:dbl[][])
            n1423 = Cluster To Array(cluster=w2774) -> (array=w2793:string[])
          }
          frame "IR-QPD + PSD + FB-QPD X position" {
            w2876 = 2  # Channel pattern
            # "convert\nADC numbers\nto volts"
            # "time average x2 the 3 psd signals (detection laser)"
            # "deinterlace 3 signals from qpds"
            n1424 = Decimate 1D Array(w2894) -> (w2893:i16[], w2892:i16[], w2829:i16[], w2830:i16[], w2839:i16[], w2836:i16[], w2833:i16[], w2864:i16[])
            n1425 = Decimate 1D Array(w2893) -> (w2891:i16[], w2878:i16[])
            n1426 = call "downsample 1D array - I16.vi"("Ave N"=2.0, "Array In"=w2839) -> ("Array Out"=w2837:i16[])  [unwired: 1 in]
            n1427 = call "downsample 1D array - I16.vi"("Ave N"=2.0, "Array In"=w2836) -> ("Array Out"=w2834:i16[])  [unwired: 1 in]
            n1428 = Decimate 1D Array(w2892) -> (w2890:i16[], w2888:i16[])
            n1429 = Decimate 1D Array(w2830) -> (w2889:i16[], w2887:i16[])
            n1430 = Decimate 1D Array(w2864) -> (w2863:i16[], w2861:i16[])
            n1431 = Decimate 1D Array(w2829) -> (w2862:i16[], w2860:i16[])
            n1432 = call "downsample 1D array - I16.vi"("Ave N"=2.0, "Array In"=w2833) -> ("Array Out"=w2831:i16[])  [unwired: 1 in]
            n1433 = Interleave 1D Arrays(w2891, w2890, w2889, w2878, w2888, w2887, w2863, w2862, w2861, w2860, w2837, w2834, w2831) -> (w2886:i16[])
            n1434 = Divide(x=w2886, y=3276.7) -> (x/y=w2885:dbl[])
            n1435 = Decimate 1D Array(w2885) -> (w2884:dbl[], w2883:dbl[], w2882:dbl[], w2881:dbl[], w2880:dbl[], w2879:dbl[], w2852:dbl[], w2850:dbl[], w2849:dbl[], w2847:dbl[], w2846:dbl[], w2845:dbl[], w2842:dbl[])
            n1436 = Divide(x=w2884, y=w2882) -> (x/y=w2868:dbl[])
            n1437 = Divide(x=w2883, y=w2882) -> (x/y=w2867:dbl[])
            n1438 = Divide(x=w2881, y=w2879) -> (x/y=w2866:dbl[])
            n1439 = Divide(x=w2880, y=w2879) -> (x/y=w2865:dbl[])
            n1440 = Divide(x=w2852, y=w2850) -> (x/y=w2851:dbl[])
            n1441 = Divide(x=w2849, y=w2847) -> (x/y=w2848:dbl[])
            n1442 = Divide(x=w2846, y=w2842) -> (x/y=w2844:dbl[])
            n1443 = Negate(x=w2842) -> (-x=w2840:dbl[])
            n1444 = Divide(x=w2845, y=w2840) -> (x/y=w2843:dbl[])
            n1445 = Bundle("T1 Y", "T1 X", "T1 Sum", "T2 Y", "T2 X", "T2 Sum", "T1 FB X", "T1 FB Sum", "T2 FB X", "T2 FB Sum", "PSD Y", "PSD X", "PSD Y Sum") -> (w2869:T43)  [unwired: 1 out]
            n1446 = Build Array(w2868, w2867, w2882, w2866, w2865, w2879, w2851, w2850, w2848, w2847, w2844, w2843, w2842) -> (w2841:dbl[][])
            n1447 = Cluster To Array(cluster=w2869) -> (array=w2877:string[])
          }
          frame "UCB Fleezers 052511" {
            w2959 = 2  # Channel pattern
            n1448 = Decimate 1D Array(w2922) -> (w2957:i16[], w2956:i16[], w2921:i16[], w2920:i16[], w2914:i16[], w2911:i16[], w2910:i16[], w2909:i16[])
            n1449 = Decimate 1D Array(w2957) -> (w2955:i16[], w2940:i16[])
            n1450 = Decimate 1D Array(w2956) -> (w2954:i16[], w2952:i16[])
            n1451 = Decimate 1D Array(w2921) -> (w2953:i16[], w2951:i16[])
            n1452 = Decimate 1D Array(w2920) -> (w2916:i16[], w2915:i16[])
            n1453 = Decimate 1D Array(w2914) -> (w2913:i16[], w2912:i16[])
            n1454 = call "downsample 1D array - I16.vi"("Ave N"=2.0, "Array In"=w2911) -> ("Array Out"=w2908:i16[])  [unwired: 1 in]
            n1455 = call "downsample 1D array - I16.vi"("Ave N"=2.0, "Array In"=w2910) -> ("Array Out"=w2907:i16[])  [unwired: 1 in]
            n1456 = call "downsample 1D array - I16.vi"("Ave N"=2.0, "Array In"=w2909) -> ("Array Out"=w2906:i16[])  [unwired: 1 in]
            n1457 = Interleave 1D Arrays(w2955, w2954, w2953, w2940, w2952, w2951, w2916, w2913, w2915, w2912, w2908, w2907, w2906) -> (w2917:i16[])
            n1458 = Divide(x=w2917, y=3276.7) -> (x/y=w2947:dbl[])
            n1459 = Decimate 1D Array(w2947) -> (w2946:dbl[], w2945:dbl[], w2944:dbl[], w2943:dbl[], w2942:dbl[], w2941:dbl[], w2905:dbl[], w2903:dbl[], w2902:dbl[], w2900:dbl[], w2899:dbl[], w2898:dbl[], w2897:dbl[])
            n1460 = Divide(x=w2946, y=w2944) -> (x/y=w2927:dbl[])
            n1461 = Divide(x=w2945, y=w2944) -> (x/y=w2926:dbl[])
            n1462 = Divide(x=w2943, y=w2941) -> (x/y=w2925:dbl[])
            n1463 = Divide(x=w2942, y=w2941) -> (x/y=w2924:dbl[])
            n1464 = Divide(x=w2905, y=w2903) -> (x/y=w2904:dbl[])
            n1465 = Divide(x=w2902, y=w2900) -> (x/y=w2901:dbl[])
            n1466 = Bundle("T1 Y", "T1 X", "T1 Sum", "T2 Y", "T2 X", "T2 Sum", "T1 FB X", "T2 FB Sum", "T2 FB X", "T2 FB Sum", "PSD Y", "PSD X", "PSD Sum") -> (w2928:T43)  [unwired: 1 out]
            n1467 = Build Array(w2927, w2926, w2944, w2925, w2924, w2941, w2904, w2903, w2901, w2900, w2899, w2898, w2897) -> (w2896:dbl[][])
            n1468 = Cluster To Array(cluster=w2928) -> (array=w2919:string[])
          }
          frame "IR-QPD + PSD + FB-QPD XY positions" {
            w3005 = 4  # Channel pattern
            # "time average x2 the 3 psd signals (detection laser)"
            # "deinterlace 3 signals from qpds"
            n1469 = Decimate 1D Array(w3029) -> (w3028:i16[], w3027:i16[], w3006:i16[], w3026:i16[], w2972:i16[], w3018:i16[], w3017:i16[], w2994:i16[])
            n1470 = Decimate 1D Array "QPD Y"(w3028) -> (w3025:i16[], w3008:i16[])
            n1471 = call "downsample 1D array - double.vi"("Ave N"=2.0, "Array In"=w3018) -> ("Array Out"=w2993:dbl[])  [unwired: 1 out]
            n1472 = call "downsample 1D array - double.vi"("Ave N"=2.0, "Array In"=w3017) -> ("Array Out"=w2992:dbl[])  [unwired: 1 out]
            n1473 = Decimate 1D Array "Feedback Sum"(w3006) -> (w2990:i16[], w2988:i16[])
            n1474 = Decimate 1D Array "Feedback Y"(w2972) -> (w2971:i16[], w2970:i16[])
            n1475 = Decimate 1D Array "Feedback X"(w2994) -> (w2991:i16[], w2989:i16[])
            n1476 = Decimate 1D Array "QPD Sum"(w3026) -> (w3023:i16[], w3021:i16[])
            n1477 = Decimate 1D Array "QPD X"(w3027) -> (w3024:i16[], w3022:i16[])
            n1478 = Interleave 1D Arrays(w3025, w3024, w3023, w3008, w3022, w3021, w2971, w2991, w2990, w2970, w2989, w2988, w2993, w2992) -> (w3016:dbl[])
            n1479 = To Word Integer(number=w3016) -> (16bit integer=w2960:i16[])
            n1480 = Divide(x=w3016, y=3276.7) -> (x/y=w3015:dbl[])
            n1481 = Decimate 1D Array(w3015) -> (w3014:dbl[], w3013:dbl[], w3012:dbl[], w3011:dbl[], w3010:dbl[], w3009:dbl[], w2967:dbl[], w2981:dbl[], w2965:dbl[], w2966:dbl[], w2979:dbl[], w2963:dbl[], w2977:dbl[], w2975:dbl[])
            n1482 = Divide(x=w3014, y=w3012) -> (x/y=w2998:dbl[])
            n1483 = Divide(x=w3013, y=w3012) -> (x/y=w2997:dbl[])
            n1484 = Divide(x=w3011, y=w3009) -> (x/y=w2996:dbl[])
            n1485 = Divide(x=w3010, y=w3009) -> (x/y=w2995:dbl[])
            n1486 = Divide(x=w2967, y=w2965) -> (x/y=w2964:dbl[])
            n1487 = Divide(x=w2981, y=w2965) -> (x/y=w2980:dbl[])
            n1488 = Divide(x=w2966, y=w2963) -> (x/y=w2962:dbl[])
            n1489 = Divide(x=w2979, y=w2963) -> (x/y=w2978:dbl[])
            n1490 = Negate(x=w2975) -> (-x=w2973:dbl[])
            n1491 = Divide(x=w2977, y=w2973) -> (x/y=w2976:dbl[])
            n1492 = Bundle("T1 Y", "T1 X", "T1 Sum", "T2 Y", "T2 X", "T2 Sum", "T1 FB Y", "T1 FB X", "T1 FB Sum", "T2 FB Y", "T2 FB X", "T2 FB Sum", "PSD X", "PSD Y Sum") -> (w2961:T44)  [unwired: 1 out]
            n1493 = Build Array(w2998, w2997, w3012, w2996, w2995, w3009, w2964, w2980, w2965, w2962, w2978, w2963, w2976, w2975) -> (w2974:dbl[][])
            n1494 = Cluster To Array(cluster=w2961) -> (array=w3007:string[])
          }
        }
      }
    }
    "AI labels" <- w2165
    n1495 = Decimate 1D Array(w2135) -> (w2163:u32[], w2099:u32[])
    n1496 = local read "DMA Update Period (s)"() -> (w2174:dbl)
    n1497 = local read "BD 1 Frequency 2 (MHz)"() -> (w2041:dbl)
    n1498 = local read "BD 1 Frequency 1 (MHz)"() -> (w2042:dbl)
    n1499 = Build Array(w2163, w2099) -> (w2241:u32[][])
    n1500 = local read "Data Period (s)"() -> (w2148:dbl)
    n1501 = Decimate 1D Array(w2049) -> (w2072:i16[], w2071:i16[], w2069:i16[], w2068:i16[])  [unwired: 9 out]
    n1502 = To Double Precision Float(number=w2241) -> (double precision float=w2242:dbl[][])
    n1503 = local read "APD Integration Time (s)"() -> (w2112:dbl)
    n1504 = Divide(x=w2072, y=w2071) -> (x/y=w2073:dbl[])
    n1505 = Divide(x=w2069, y=w2068) -> (x/y=w2070:dbl[])
    n1506 = feedback #1(0.0) -> (w2086:dbl)
    n1507 = Add(x=w2174, y=w2086) -> (x+y=w2281:dbl)
